vi "DM_Control_Main_V2.vi"() -> ()   [LabVIEW 2014]
uses:
  Controls/Pixel Scan Parameters.ctl
  Controls/MirrorModes.ctl
  Controls/Standard Action.ctl
  <vilib>/Analysis/baseanly.llb/Mean (DBL).vi
  <vilib>/Utility/file.llb/Write To Spreadsheet File (DBL).vi
  <vilib>/Utility/file.llb/Read From Spreadsheet File (DBL).vi
  <vilib>/Analysis/NI_AALBase.lvlib
panel:
  in  "Load Flat":bool
  in  "Apply Zero":bool
  in  "Load V Map":bool
  in  "Save V Map":bool
  in  "Apply Flat":bool
  in  "Center Bias":bool
  in  "Exit":bool
  in  "Mirror Tab":enum32{"Mirror Modes", "Scan Pixels"}(tab)
  in  "Clear Modes":bool
  in  "Mirror Modes":T1
  in  "Load Modes":bool
  in  "Save Modes":bool
  in  "Scan Modes":bool
  in  "Pixel Scan Parameters":T2={"Scan Start Pixel"=1, "Scan End Pixel"=1, "Pixel Start Value (-1 to 1)"=-0.5, "Pixel End Value (-1 to 1)"=0.5, "Number of Steps"=0.1}
  in  "Start Pixel Scan":bool
  out "Pixel Map (-1 to 1)":dbl[][](graph)
  # "Mode"
  # "Amount (nm)"
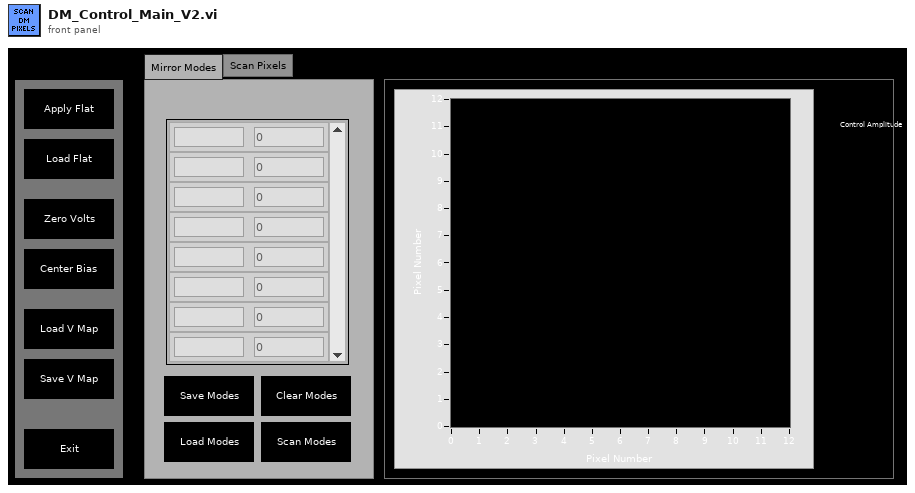
[diagram p1: front panel]
types:
  T1 = typedef "MirrorModes.ctl" = cluster{"Mode":string, "Amplitude":dbl}[]
  T2 = typedef "Pixel Scan Parameters.ctl" = cluster{"Scan Start Pixel":i32, "Scan End Pixel":i32, "Pixel Start Value (-1 to 1)":dbl, "Pixel End Value (-1 to 1)":dbl, "Number of Steps":dbl}
  T3 = typedef "Standard Action.ctl" = enum16{"Read", "Write"}
  T4 = enum16{"Start Scan", "Reset Counter", "Write DM", "Get Image", "Update Count", "Exit"}
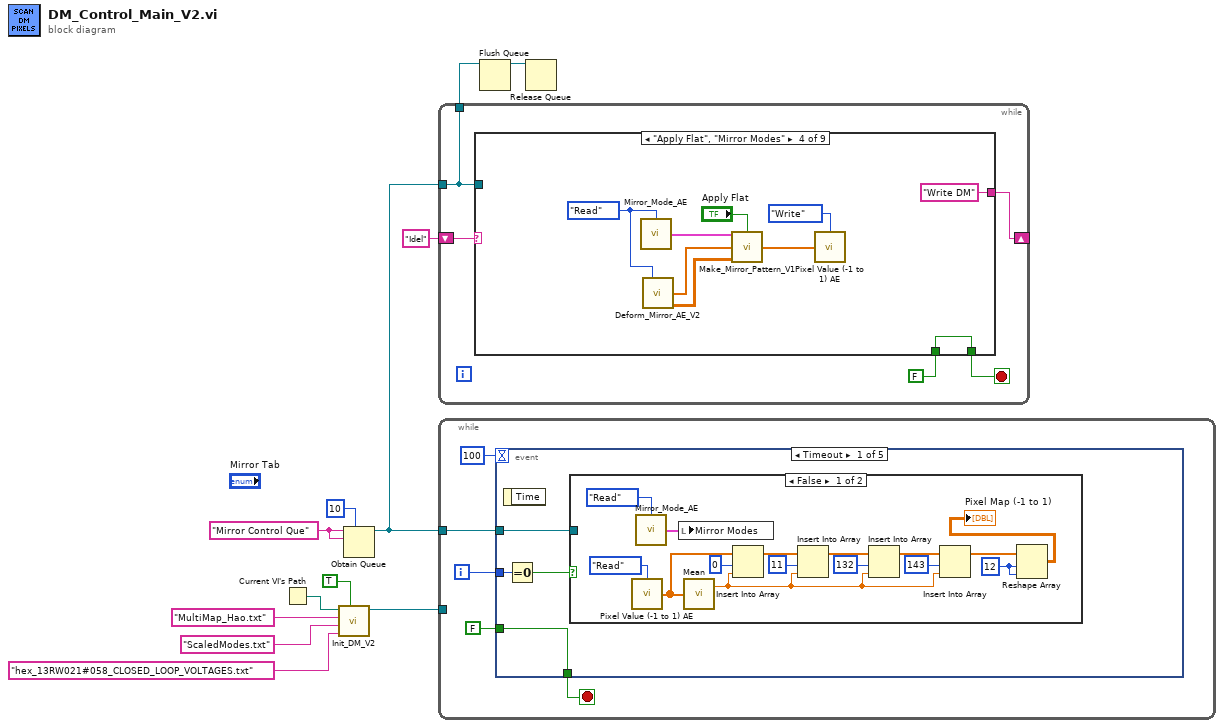
[diagram p0: block diagram]
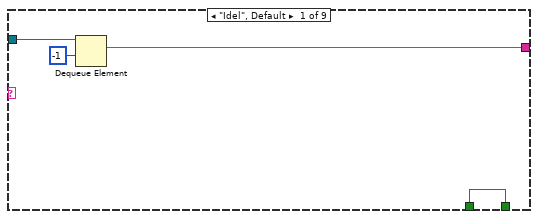
[diagram p2: hidden frame]
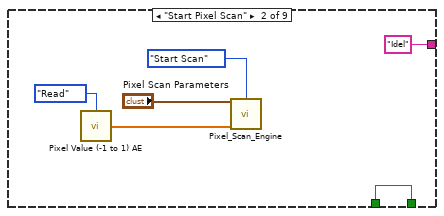
[diagram p3: hidden frame]
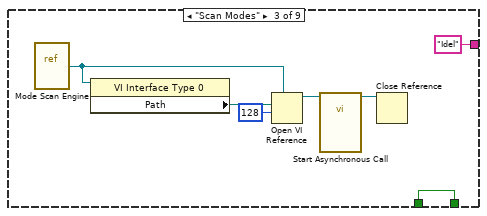
[diagram p4: hidden frame]
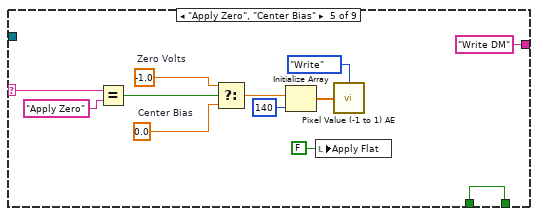
[diagram p5: hidden frame]
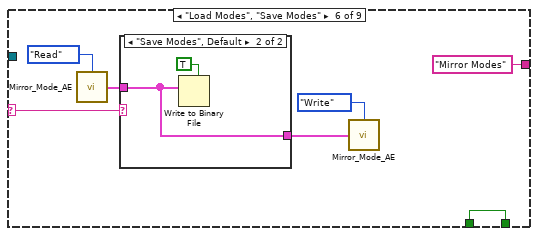
[diagram p6: hidden frame]
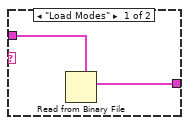
[diagram p7: hidden frame]
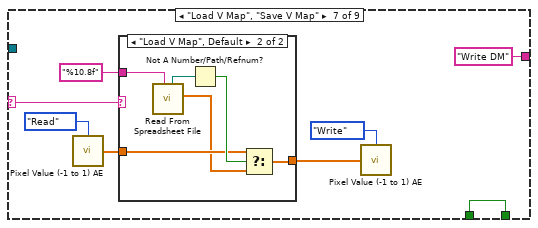
[diagram p8: hidden frame]
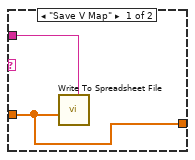
[diagram p9: hidden frame]
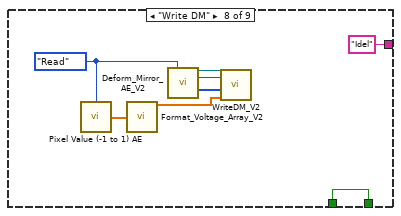
[diagram p10: hidden frame]
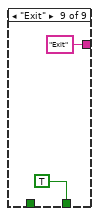
[diagram p11: hidden frame]
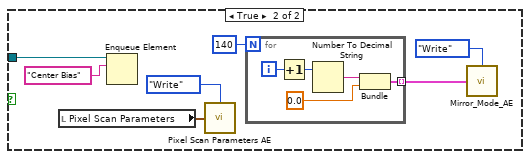
[diagram p12: hidden frame]
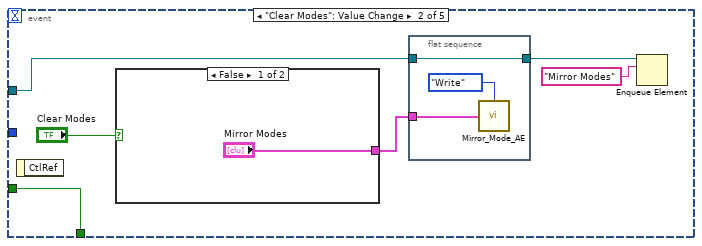
[diagram p13: hidden frame]
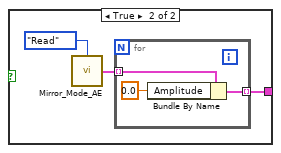
[diagram p14: hidden frame]
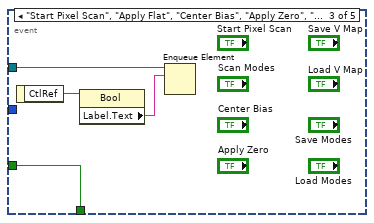
[diagram p15: hidden frame]
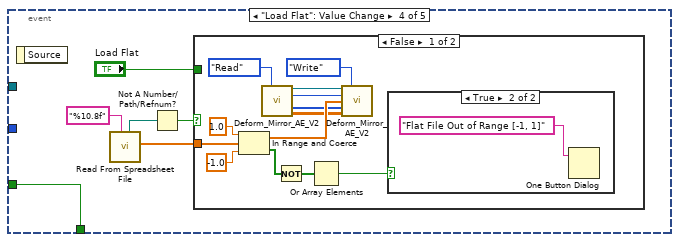
[diagram p16: hidden frame]
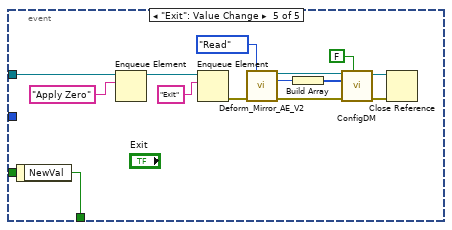
[diagram p19: hidden frame]
diagram:
  w12 = "Mirror Control Que" ("name (unnamed)")
  n1 = Current VI's Path() -> (path=w4:path)
  n2 = call "Init_DM_V2.vi"("BM Flat"=TRUE, "BM Flat File"="hex_13RW021#058_CLOSED_LOOP_VOLTAGES.txt" ("name or relative path"), "Mirror Modes File"="ScaledModes.txt" ("name or relative path"), "DM Mapping File"="MultiMap_Hao.txt" ("name or relative path"), "Base File Path"=w4) -> ("reference out"=w10:refnum<k7>)  [unwired: 6 in]
  n3 = Obtain Queue(max queue size (-1, unlimited)=10, name (unnamed)=w12, element data type=w12) -> (queue out=w6:refnum<queue>)  [unwired: 2 in, 2 out]
  n4 = while {
    tunnel: w6 -> [w13]
    shift-right: [w17] -> _
    shift-left: "Idel" ("name (unnamed)") -> [w16]
    tunnel: [w13] -> w9
    stop <- w15 stop-if-true
    n5 = case shown="\"Apply Flat\", \"Mirror Modes\"" w16 {
      selector: w16 -> [_ _ _ _ w50 w58 w73 _ _]
      tunnel: w13 -> [w21 _ _ _ _ _ _ _ _]
      tunnel: [w19 "Idel" ("name (unnamed)") "Idel" ("name (unnamed)") "Write DM" ("name (unnamed)") "Write DM" ("name (unnamed)") "Mirror Modes" ("name (unnamed)") "Write DM" ("name (unnamed)") "Idel" ("name (unnamed)") "Exit" ("name (unnamed)")] -> w17
      tunnel: [w18 w27 w34 w42 w55 w62 w74 w90 TRUE] -> w15
      tunnel: FALSE -> [w18 w27 w34 w42 w55 w62 w74 w90 _]
      frame "Idel", Default {
        n6 = Dequeue Element(queue=w21, timeout in ms (-1)=-1) -> (element=w19:string)  [unwired: 1 in, 3 out]
      }
      frame "Start Pixel Scan" {
        n7 = call "Pixel Value (-1 to 1) AE.vi"("Action"=Standard_Action."Read") -> ("Pixel Value (-1 to 1) Out"=w25:dbl[])  [unwired: 14 in]
        n8 = call "Pixel_Scan_Engine.vi"("Pixel Scan Parameters In"="Pixel Scan Parameters", "Action"=T4."Start Scan", "Initial Pixel Values (-1 to 1)"=w25) -> ()  [unwired: 13 in]
      }
      frame "Scan Modes" {
        n9 = vi-ref "Mode Scan Engine.vi"() -> (w28:refnum<vi>)
        n10 = property class="VI Interface Type 0"(reference=w28) -> ("Path"=w29:path)  [unwired: 1 in, 2 out]
        n11 = Open VI Reference(type specifier VI Refnum (for type only)=w28, vi path=w29, options=128) -> (vi reference=w31:refnum<vi>)  [unwired: 3 in, 1 out]
        n12 = call-by-ref "Start Asynchronous Call"(reference=w31) -> (reference out=w32:refnum<vi>)  [unwired: 17 in, 1 out]
        n13 = Close Reference(reference=w32) -> ()  [unwired: 1 in, 1 out]
      }
      frame "Apply Flat", "Mirror Modes" {
        w36 = Standard_Action."Read" ("Action")
        n14 = call "Mirror_Mode_AE.vi"("Action"=w36) -> ("Mirror Modes Out"=w39:T1)  [unwired: 14 in]
        n15 = call "Deform_Mirror_AE_V2.vi"("Action"=w36) -> ("Flat Files Out"=w40:dbl[], "Mode Matrix Out"=w41:dbl[][])  [unwired: 10 in, 3 out]
        n16 = call "Make_Mirror_Pattern_V1.vi"("Mirror Modes In"=w39, "Flat On?"="Apply Flat", "Flat File In"=w40, "Mirror Modes Array"=w41) -> ("Pixel Value U (-1 to 1)"=w38:dbl[])  [unwired: 11 in]
        n17 = call "Pixel Value (-1 to 1) AE.vi"("Action"=Standard_Action."Write", "Pixel Value (-1 to 1)"=w38) -> ()  [unwired: 13 in, 1 out]
      }
      frame "Apply Zero", "Center Bias" {
        w46 = -1.0  # Zero Volts
        w48 = 0.0  # Center Bias
        n18 = Equal?(x=w50, y="Apply Zero") -> (x = y?=w49:bool)
        n19 = Select(t=w46, s=w49, f=w48) -> (s? t:f=w47:dbl)
        n20 = Initialize Array(w47, 140 ("dimension size")) -> (w53:dbl[])
        n21 = local write "Apply Flat"(FALSE ("Apply Flat")) -> ()
        n22 = call "Pixel Value (-1 to 1) AE.vi"("Action"=Standard_Action."Write", "Pixel Value (-1 to 1)"=w53) -> ()  [unwired: 13 in, 1 out]
      }
      frame "Load Modes", "Save Modes" {
        n23 = call "Mirror_Mode_AE.vi"("Action"=Standard_Action."Read") -> ("Mirror Modes Out"=w57:T1)  [unwired: 14 in]
        n24 = case shown="\"Save Modes\", Default" w58 {
          tunnel: w57 -> [w64 w65]
          tunnel: [w63 w65] -> w56
          frame "Load Modes" {
            n25 = Read from Binary File(5:w64) -> (2:w63:T1)  [unwired: 5 in, 3 out]
          }
          frame "Save Modes", Default {
            n26 = Write to Binary File(data=w65, 5:TRUE ("prepend array or string size? (T)")) -> ()  [unwired: 4 in, 3 out]
          }
        }
        n27 = call "Mirror_Mode_AE.vi"("Action"=Standard_Action."Write", "Mirror Modes In"=w56) -> ()  [unwired: 13 in, 1 out]
      }
      frame "Load V Map", "Save V Map" {
        n28 = call "Pixel Value (-1 to 1) AE.vi"("Action"=Standard_Action."Read") -> ("Pixel Value (-1 to 1) Out"=w71:dbl[])  [unwired: 14 in]
        n29 = case shown="\"Load V Map\", Default" w73 {
          tunnel: w71 -> [w75 w79]
          tunnel: "%10.8f" -> [w76 w82]
          tunnel: [w75 w77] -> w67
          frame "Save V Map" {
            n30 = call-poly <vilib>:"Write To Spreadsheet File.vi"("format (%.3f)"=w76, "1D data"=w75) -> ()  [unwired: 6 in, 1 out]
          }
          frame "Load V Map", Default {
            n31 = call-poly <vilib>:"Read From Spreadsheet File.vi"("format (%.3f)"=w82) -> ("first row"=w78:dbl[], "new file path (Not A Path if cancelled)"=w81:path)  [unwired: 6 in, 3 out]
            n32 = Not A Number/Path/Refnum?(number/path/refnum=w81) -> (NaN/Path/Refnum?=w80:bool)
            n33 = Select(t=w79, s=w80, f=w78) -> (s? t:f=w77:dbl[])
          }
        }
        n34 = call "Pixel Value (-1 to 1) AE.vi"("Action"=Standard_Action."Write", "Pixel Value (-1 to 1)"=w67) -> ()  [unwired: 13 in, 1 out]
      }
      frame "Write DM" {
        w88 = Standard_Action."Read" ("Action")
        n35 = call "Pixel Value (-1 to 1) AE.vi"("Action"=w88) -> ("Pixel Value (-1 to 1) Out"=w87:dbl[])  [unwired: 14 in]
        n36 = call "Format_Voltage_Array_V2.vi"("Pixel Level (-1 to 1)"=w87) -> ("Voltage Array (Volts)"=w83:dbl[])  [unwired: 13 in, 1 out]
        n37 = call "Deform_Mirror_AE_V2.vi"("Action"=w88) -> ("Refnum Out"=w86:refnum<k7>, "IDs Out"=w85:i32, "Multi Map Data Out"=w84:i32[])  [unwired: 10 in, 2 out]
        n38 = call "WriteDM_V2.vi"("reference in"=w86, "nDevId"=w85, "MultiDM  Mapping"=w84, "Voltage Array in"=w83) -> ()  [unwired: 2 in, 2 out]
      }
      frame "Exit" {
      }
    }
  }
  n39 = while {
    tunnel: w6 -> [w93]
    tunnel: w10 -> [_]
    i -> [w94]
    stop <- w97 stop-if-true
    n40 = event shown="[0] Timeout" {
      selector: _ -> [_ _ _ _ _]
      dyn-events: _ -> [_ _ _ _ _]
      timeout: 100 -> [_ _ _ _ _]
      tunnel: [w101 w134 w148 w154 w181] -> w97
      tunnel: FALSE -> [w101 w134 w148 w154 _]
      tunnel: w94 -> [w100 _ _ _ _]
      tunnel: w93 -> [w98 w133 w147 _ w179]
      event Timeout {
        n41 = event-data() -> ()  [unwired: 1 in, 1 out]
        n42 = Equal To 0?(x=w100) -> (x = 0?=w99:bool)
        n43 = case shown="False" w99 {
          tunnel: w98 -> [_ w123]
          frame False {
            w115 = 12 ("dimension size")
            n44 = call "Pixel Value (-1 to 1) AE.vi"("Action"=Standard_Action."Read") -> ("Pixel Value (-1 to 1) Out"=w116:dbl[])  [unwired: 14 in]
            n45 = call "Mirror_Mode_AE.vi"("Action"=Standard_Action."Read") -> ("Mirror Modes Out"=w103:T1)  [unwired: 14 in]
            n46 = local write "Mirror Modes"(w103) -> ()
            n47 = call-poly <vilib>:"Mean.vi"("X"=w116) -> ("mean"=w113:dbl)  [unwired: 1 out]
            n48 = Insert Into Array(array=w116, index=0, new element=w113) -> (w108:dbl[])
            n49 = Insert Into Array(array=w108, index=11, new element=w113) -> (w110:dbl[])
            n50 = Insert Into Array(array=w110, index=132, new element=w113) -> (w112:dbl[])
            n51 = Insert Into Array(array=w112, index=143, new element=w113) -> (w105:dbl[])
            n52 = Reshape Array(w105, w115, w115) -> (→"Pixel Map (-1 to 1)":dbl[][])
          }
          frame True {
            n53 = local read "Pixel Scan Parameters"() -> (w120:T2)
            n54 = Enqueue Element(queue=w123, element="Center Bias") -> ()  [unwired: 2 in, 3 out]
            n55 = call "Pixel Scan Parameters AE.vi"("Action"=enum16{"Write", "Read"}."Write", "Pixel Scan Parameters"=w120) -> ()  [unwired: 13 in, 1 out]
            n56 = for {
              N: 140 -> [_]
              tunnel: [w124] -> w117 mode=indexing
              i -> [w128]
              n57 = Increment(x=w128) -> (x+1=w127:i32)
              n58 = Number To Decimal String(number=w127) -> (decimal integer string=w126:string)  [unwired: 1 in]
              n59 = Bundle(w126, 0.0) -> (w124:cluster{string, dbl})  [unwired: 1 in]
            }
            n60 = call "Mirror_Mode_AE.vi"("Action"=Standard_Action."Write", "Mirror Modes In"=w117) -> ()  [unwired: 13 in, 1 out]
          }
        }
      }
      event "Clear Modes": Value Change {
        n61 = event-data() -> ()  [unwired: 1 in, 1 out]
        n62 = case shown="False" "Clear Modes" {
          tunnel: ["Mirror Modes" w136] -> w129
          frame False {
          }
          frame True {
            n63 = call "Mirror_Mode_AE.vi"("Action"=Standard_Action."Read") -> ("Mirror Modes Out"=w138:T1)  [unwired: 14 in]
            n64 = for {
              tunnel: w138 -> [w141] mode=indexing
              tunnel: [w139] -> w136 mode=indexing
              n65 = Bundle By Name(cluster=w141, "Amplitude"=0.0) -> (w139:cluster{"Mode":string, "Amplitude":dbl})
            }
          }
        }
        n66 = flat-sequence {
          tunnel: w129 -> [w143]
          tunnel: w133 -> [w142]
          tunnel: [w142] -> w131
          frame #0 {
            n67 = call "Mirror_Mode_AE.vi"("Action"=Standard_Action."Write", "Mirror Modes In"=w143) -> ()  [unwired: 13 in, 1 out]
          }
        }
        n68 = Enqueue Element(queue=w131, element="Mirror Modes") -> ()  [unwired: 2 in, 3 out]
      }
      event "Start Pixel Scan", "Apply Flat", "Center Bias", "Apply Zero", "Save V Map", "Save Modes", "Load Modes", "Load V Map", "Scan Modes": Value Change {
        n69 = event-data() -> ("CtlRef"=w146:refnum<vi>)  [unwired: 1 in]
        n70 = property class="Bool"(reference=w146) -> ("Label.Text"=w145:string)  [unwired: 1 in, 2 out]
        n71 = Enqueue Element(queue=w147, element=w145) -> ()  [unwired: 2 in, 3 out]
      }
      event "Load Flat": Value Change {
        n72 = event-data() -> ()  [unwired: 1 in, 1 out]
        n73 = call-poly <vilib>:"Read From Spreadsheet File.vi"("format (%.3f)"="%10.8f") -> ("first row"=w150:dbl[], "new file path (Not A Path if cancelled)"=w152:path)  [unwired: 6 in, 3 out]
        n74 = Not A Number/Path/Refnum?(number/path/refnum=w152) -> (NaN/Path/Refnum?=w151:bool)
        n75 = case shown="False" w151 {
          tunnel: w150 -> [w167 _]
          tunnel: "Load Flat" -> [_ _]
          frame False {
            n76 = In Range and Coerce(upper limit=1.0, x=w167, lower limit=-1.0) -> (coerced(x)=w160:dbl[], In Range?=w164:bool[])
            n77 = call "Deform_Mirror_AE_V2.vi"("Action"=Standard_Action."Read") -> ("Refnum Out"=w156:refnum<k7>, "IDs Out"=w157:i32, "Multi Map Data Out"=w158:i32[], "Mode Matrix Out"=w159:dbl[][])  [unwired: 10 in, 1 out]
            n78 = Not(x=w164) -> (.not. x?=w163:bool[])
            n79 = Or Array Elements(Boolean array=w163) -> (logical OR=w155:bool)
            n80 = call "Deform_Mirror_AE_V2.vi"("Refnum In"=w156, "Action"=Standard_Action."Write", "IDs In"=w157, "Flat Files In"=w160, "Multi Map Data In"=w158, "Mode Matrix"=w159) -> ()  [unwired: 5 in, 5 out]
            n81 = case shown="True" w155 {
              frame False {
              }
              frame True {
                n82 = One Button Dialog(message="Flat File Out of Range [-1, 1]") -> ()  [unwired: 1 in, 1 out]
              }
            }
          }
          frame True {
          }
        }
      }
      event "Exit": Value Change {
        n83 = event-data() -> ("NewVal"=w181:bool)  [unwired: 1 in]
        n84 = Enqueue Element(queue=w179, element="Apply Zero") -> (queue out=w178:refnum<queue>)  [unwired: 2 in, 2 out]
        n85 = Enqueue Element(queue=w178, element="Exit") -> (error out=w170:errorcluster)  [unwired: 2 in, 2 out]
        n86 = call "Deform_Mirror_AE_V2.vi"("Action"=Standard_Action."Read") -> ("Refnum Out"=w173:refnum<k7>, "IDs Out"=w174:i32)  [unwired: 10 in, 3 out]
        n87 = Build Array(w174) -> (w175:i32[])
        n88 = call "ConfigDM.vi"("High Voltage"=FALSE, "error in (no error)"=w170, "Dev IDs"=w175, "Automation Refnum in"=w173) -> ("error out"=w169:errorcluster, "Automation Refnum out"=w172:refnum<k7>)  [unwired: 6 in]
        n89 = Close Reference(reference=w172, error in (no error)=w169) -> ()  [unwired: 1 out]
      }
    }
  }
  n90 = Flush Queue(queue=w9) -> (queue out=w8:refnum<queue>)  [unwired: 1 in, 2 out]
  n91 = Release Queue(queue=w8) -> ()  [unwired: 2 in, 3 out]
